vi "MK210_DO_Write.vi"(8 "Error In":errorcluster, 9 "Button":bool=TRUE, 10 "n of on":u8=1, 11 "Sustain":string="\u0001\u0003\u0002\u0000ýø\u0004") -> (0 "Error Out":errorcluster, 2 "BIN OUT":string, 3 "concatenated string":string)   [LabVIEW 2018]
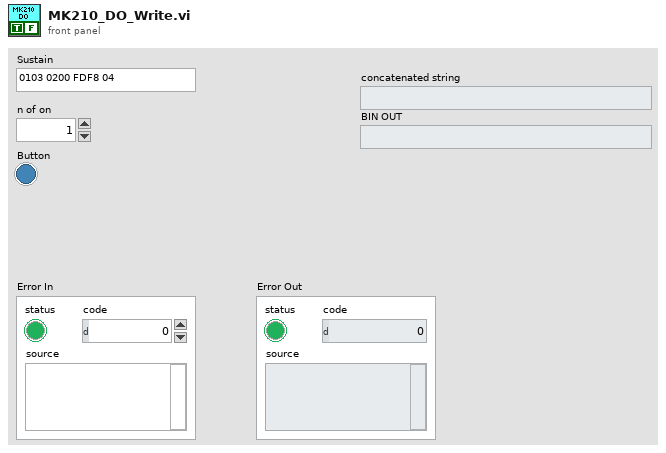
[diagram p1: front panel]
types:
  T1 = typedef "MLLC_Error.ctl" = errorcluster
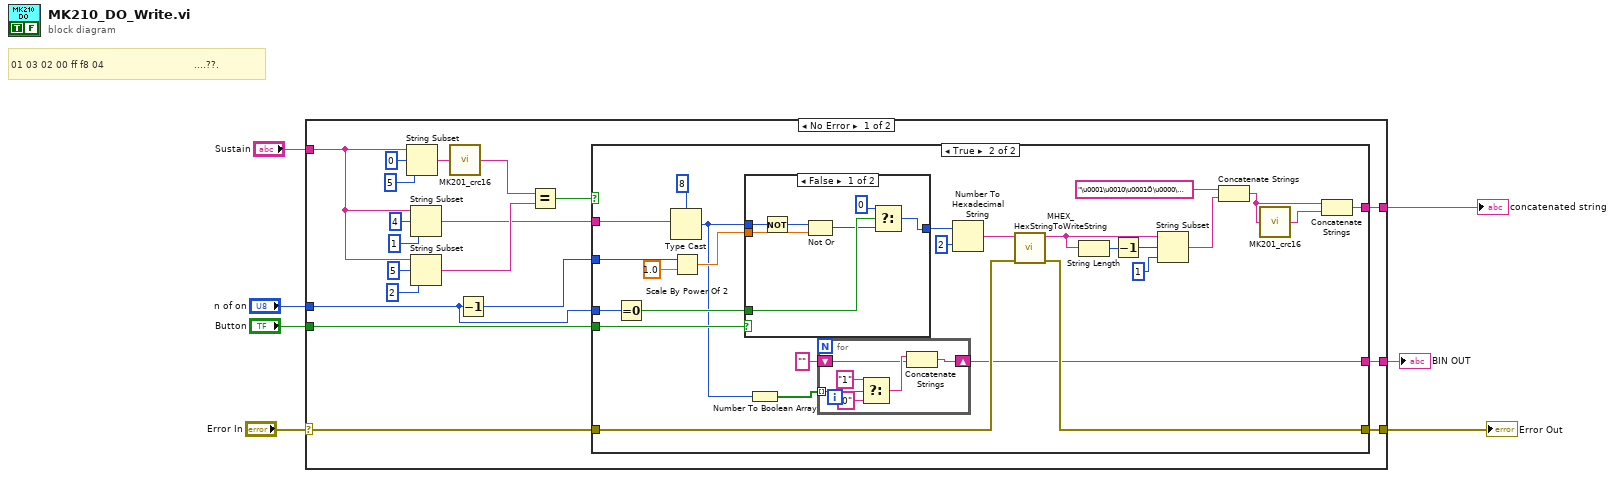
[diagram p0: block diagram]
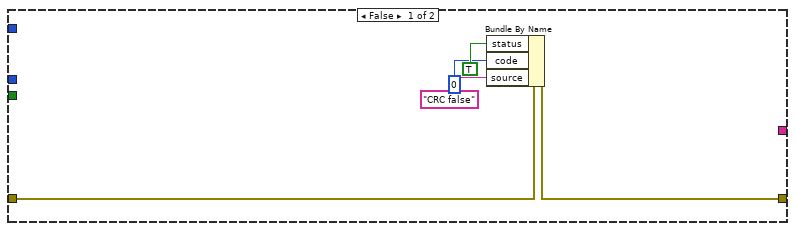
[diagram p2: hidden frame]
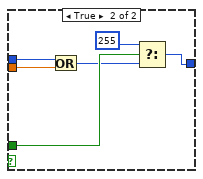
[diagram p3: hidden frame]
diagram:
  # "01 03 02 00 ff f8 04                              ....??."
  n1 = case shown="No Error" "Error In" {
    selector: "Error In" -> [w12 w77]
    tunnel: "Sustain" -> [w20 _]
    tunnel: "n of on" -> [w10 _]
    tunnel: [w14 _] -> w5
    tunnel: "Button" -> [w13 _]
    tunnel: [w11 w77] -> w2
    tunnel: [w9 _] -> w1
    frame No Error {
      n2 = String Subset(string=w20, offset (0)=0, length (rest)=5 ("length (rest)")) -> (substring=w19:string)
      n3 = String Subset(string=w20, offset (0)=4, length (rest)=1 ("length (rest)")) -> (substring=w16:string)
      n4 = String Subset(string=w20, offset (0)=5, length (rest)=2 ("length (rest)")) -> (substring=w17:string)
      n5 = call "MK201_crc16.vi"("message"=w19) -> ("CRC16"=w18:string)  [unwired: 4 in]
      n6 = Decrement(x=w10) -> (x-1=w15:u8)
      n7 = Equal?(x=w18, y=w17) -> (x = y?=w8:bool)
      n8 = case shown="True" w8 {
        tunnel: w16 -> [_ w57]
        tunnel: w15 -> [_ w38]
        tunnel: [_ w47] -> w14
        tunnel: w13 -> [_ w46]
        tunnel: w12 -> [w31 w40]
        tunnel: [w30 w39] -> w11
        tunnel: w10 -> [_ w37]
        tunnel: [_ w32] -> w9
        frame False {
          n9 = Bundle By Name(cluster=w31, "status"=TRUE, "code"=0, "source"="CRC false") -> (w30:errorcluster)
        }
        frame True {
          n10 = Equal To 0?(x=w37) -> (x = 0?=w36:bool)
          n11 = Type Cast(type=u8 8, x=w57) -> (*(type *) &x=w35:u8)
          n12 = Scale By Power Of 2(n=w38, x=1.0) -> (x*2^n=w52:dbl)
          n13 = case shown="False" w46 {
            tunnel: w35 -> [w70 w76]
            tunnel: [w64 w71] -> w53
            tunnel: w52 -> [w68 w75]
            tunnel: w36 -> [w66 w74]
            frame False {
              n14 = Not(x=w70) -> (.not. x?=w69:u8)
              n15 = Not Or(1:w68, 2:w69) -> (0:w65:i32)
              n16 = Select(t=0, s=w66, f=w65) -> (s? t:f=w64:i32)
            }
            frame True {
              n17 = Or(x=w76, y=w75) -> (x .or. y?=w73:i32)
              n18 = Select(t=255, s=w74, f=w73) -> (s? t:f=w71:i32)
            }
          }
          n19 = Number To Boolean Array(number=w35) -> (Boolean array=w34:bool[])
          n20 = for {
            tunnel: w34 -> [w63] mode=indexing
            shift-right: [w60] -> w32
            shift-left: "" -> [w58]
            n21 = Select(t="1", s=w63, f="0") -> (s? t:f=w59:string)
            n22 = Concatenate Strings(w59, w58) -> (w60:string)
          }
          n23 = Number To Hexadecimal String(1:i16 2 ("width (-)"), 2:w53) -> (0:w55:string)
          n24 = call "MHEX_HexStringToWriteString.vi"("Error in (no error)"=w40, "STRING HEX"=w55) -> ("Error out"=w39:T1, "String out"=w45:string)  [unwired: 6 in, 2 out]
          n25 = String Length(string=w45) -> (length=w43:i32)
          n26 = Decrement(x=w43) -> (x-1=w42:i32)
          n27 = String Subset(string=w45, offset (0)=w42, length (rest)=1 ("length (rest)")) -> (substring=w41:string)
          n28 = Concatenate Strings("\u0001\u0010\u0001Ö\u0000\u0001\u0002\u0000", w41) -> (w49:string)
          n29 = call "MK201_crc16.vi"("message"=w49) -> ("CRC16"=w48:string)  [unwired: 4 in]
          n30 = Concatenate Strings(w49, w48) -> (w47:string)
        }
      }
    }
    frame Error {
    }
  }
  "concatenated string" <- w5
  "Error Out" <- w2
  "BIN OUT" <- w1
